vi "ClearError.vi"(4 "Clear Mode(0:Clear All)":enum16{"Clear All", "Clear Specific"}(ring), 6 "Code to Clear(0)":i32, 8 "Show Error Dialog?(F:No)":bool, 9 "error in (no error)":errorcluster) -> (1 "error out":errorcluster)   [LabVIEW 2020]
panel:
  # "Inputs"
  # "Outputs"
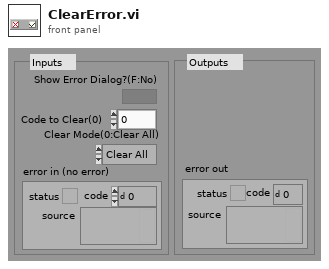
[diagram p1: front panel]
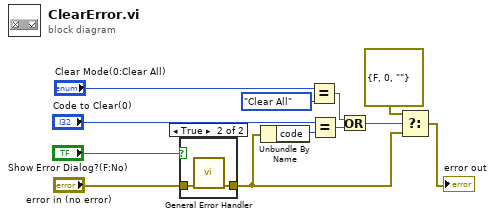
[diagram p0: block diagram]
diagram:
  n1 = case shown="True" "Show Error Dialog?(F:No)" {
    tunnel: [w13 w15] -> w8
    tunnel: "error in (no error)" -> [w13 w14]
    frame False {
    }
    frame True {
      n2 = call <vilib>:"General Error Handler.vi"("error in (no error)"=w14) -> ("error out"=w15:errorcluster)  [unwired: 10 in, 4 out]
    }
  }
  n3 = Unbundle By Name(w8) -> ("code"=w7:i32)
  n4 = Equal?(x="Clear Mode(0:Clear All)", y=enum16{"Clear All", "Clear Specific"}."Clear All" ("Clear Mode(0:Clear All)")) -> (x = y?=w11:bool)
  n5 = Equal?(x="Code to Clear(0)", y=w7) -> (x = y?=w10:bool)
  n6 = Or(x=w11, y=w10) -> (x .or. y?=w9:bool)
  n7 = Select(t=errorcluster {"status"=FALSE, "code"=0, "source"=""}, s=w9, f=w8) -> (s? t:f=→"error out":errorcluster)
